vi "Configure Remote Terminal 2.vi"(8 "error in (no error)":errorcluster) -> (0 "error out":errorcluster, 3 "Remote Terminal":refnum<class "Remote Terminal.lvclass">)   [LabVIEW 2016, in "BCI-1553 RealTime API Examples.lvlib"]
uses:
  BCI-1553 RealTime API Examples.lvlib
  <vilib>/Bloomy/BCI-1553 Driver/RealTime/Remote Terminal/Remote Terminal.lvclass
  <vilib>/Bloomy/BCI-1553 Driver/RealTime/Frames & Messages/TypeDefs/Command Terminal Address.ctl
  <vilib>/Bloomy/BCI-1553 Driver/RealTime/Frames & Messages/TypeDefs/Command Type.ctl
  <vilib>/Bloomy/BCI-1553 Driver/RealTime/Frames & Messages/TypeDefs/Command SubAddress.ctl
  <vilib>/Bloomy/BCI-1553 Driver/RealTime/Frames & Messages/TypeDefs/Command Word Count.ctl
  <vilib>/Bloomy/BCI-1553 Driver/RealTime/Remote Terminal/TypeDefs/RT Configuration.ctl
  <vilib>/Bloomy/BCI-1553 Driver/RealTime/Remote Terminal/TypeDefs/RT-RT Timeout.ctl
  <vilib>/Bloomy/BCI-1553 Driver/RealTime/Remote Terminal/TypeDefs/Mode Code 17 Sync Configuration.ctl
  <vilib>/Bloomy/BCI-1553 Driver/RealTime/Remote Terminal/TypeDefs/RT Timetag Configuration.ctl
  <vilib>/Bloomy/BCI-1553 Driver/RealTime/BCI-1553 API.lvlib
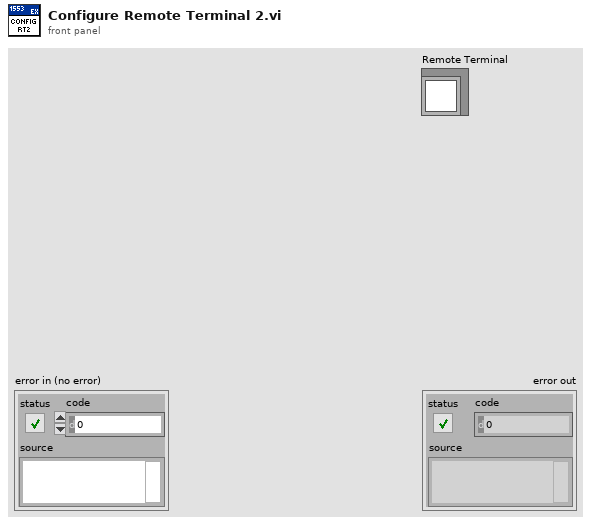
[diagram p1: front panel]
types:
  T1 = typedef "BCI-1553 API.lvlib/Remote Terminal.lvclass/RT Timetag Configuration.ctl" = enum16{"Disabled", "2us", "4us", "8us", "16us", "32us", "64us"}
  T2 = typedef "BCI-1553 API.lvlib/Remote Terminal.lvclass/RT-RT Timeout.ctl" = enum16{"57us", "62us", "100us", "180us"}
  T3 = typedef "BCI-1553 API.lvlib/Remote Terminal.lvclass/RT Configuration.ctl" = cluster{"RT-RT Timeout":T2, "Inhibit Bus A":bool, "Inhibit Bus B":bool, "Broadcast CMD Invalid":bool, "UnDef MCs Invalid":bool, "Notice 2 Data Storage":bool, "SMCP":bool, "Temp RX Buffer":bool, "Alt BIT Enable":bool, "Auto Bus Shutdown":bool, "MC 16 SR Reset":bool, "MC 17 Sync":T4, "MC 8 Reset":bool, "Remote Terminal Timetag Config":T1}
  T4 = typedef "BCI-1553 API.lvlib/Remote Terminal.lvclass/Mode Code 17 Sync Configuration.ctl" = enum16{"Sync if Bit 0 = 1", "Sync if Bit 0 = 0", "Sync Unconditionally"}
  T5 = typedef "BCI-1553 API.lvlib/Command Word Count.ctl" = enum16{"1", "2", "3", "4", "5", "6", "7", "8", "9", "10", "11", "12", "13", "14", "15", "16", "17", "18", "19", "20", "21", "22", "23", "24", "25", "26", "27", "28", "29", "30", "31", "32"}
  T6 = typedef "BCI-1553 API.lvlib/Command SubAddress.ctl" = enum16{"Mode Code", "1", "2", "3", "4", "5", "6", "7", "8", "9", "10", "11", "12", "13", "14", "15", "16", "17", "18", "19", "20", "21", "22", "23", "24", "25", "26", "27", "28", "29", "30"}
  T7 = typedef "BCI-1553 API.lvlib/Command Type.ctl" = enum16{"Transmit", "Receive"}
  T8 = typedef "BCI-1553 API.lvlib/Command Terminal Address.ctl" = enum16{"0", "1", "2", "3", "4", "5", "6", "7", "8", "9", "10", "11", "12", "13", "14", "15", "16", "17", "18", "19", "20", "21", "22", "23", "24", "25", "26", "27", "28", "29", "30", "Broadcast"}
  T9 = typedef "BCI-1553 API.lvlib/Remote Terminal.lvclass/RT Command Config.ctl" = cluster{"Command Type":T7, "SubAddress":T6, "Word Count\\Mode Code":T5, "Initial Data":u16[], "Data Fields":T10[]}
  T10 = typedef "BCI-1553 API.lvlib/Simplified Parameter Data Table.ctl" = cluster{"Parameter Name":string, "Base Word":u16, "Scaling Info":T11}
  T11 = typedef "BCI-1553 API.lvlib/Scaling Information.ctl" = cluster{"Bit Offset":i32, "Bit Count":i32, "LSB Resolution":dbl, "2's Complement":bool, "Big Endian":bool, "Sign Bit":bool}
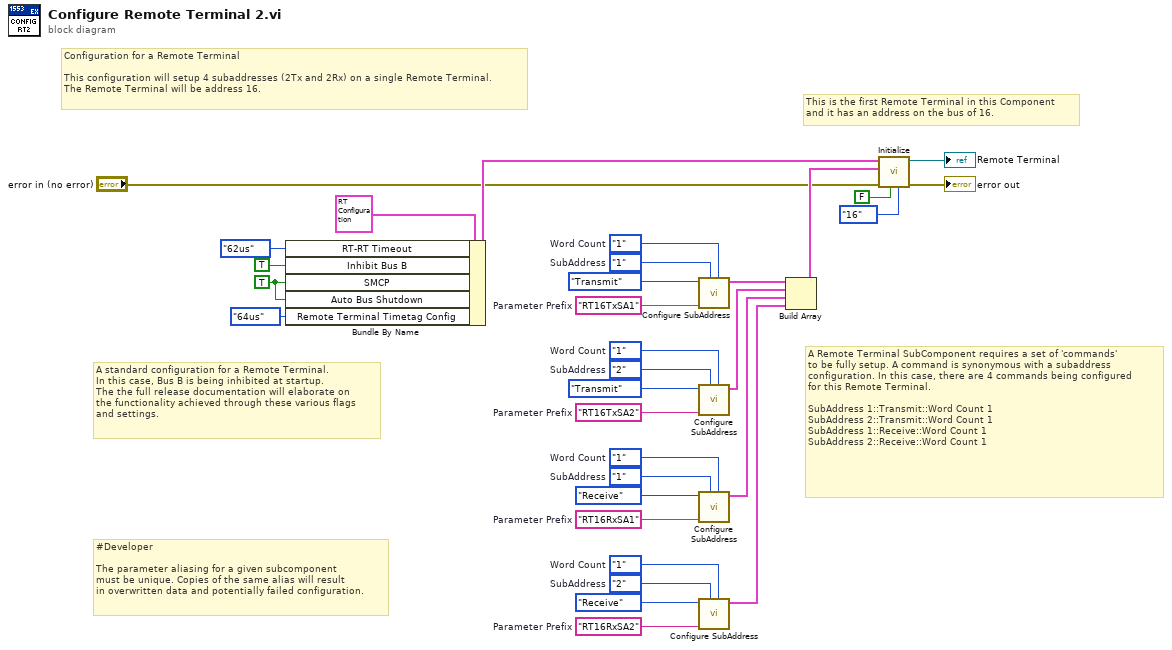
[diagram p0: block diagram]
diagram:
  w2 = TRUE ("SMCP")
  w16 = Command_Word_Count."1"  # Word Count
  w15 = Command_SubAddress."2"  # SubAddress
  w18 = Command_Word_Count."1"  # Word Count
  w17 = Command_SubAddress."1"  # SubAddress
  w19 = Command_Word_Count."1"  # Word Count
  w20 = Command_SubAddress."2"  # SubAddress
  w21 = "RT16RxSA2"  # Parameter Prefix
  w22 = "RT16RxSA1"  # Parameter Prefix
  w23 = "RT16TxSA2"  # Parameter Prefix
  w24 = "RT16TxSA1"  # Parameter Prefix
  w25 = Command_Word_Count."1"  # Word Count
  w26 = Command_SubAddress."1"  # SubAddress
  # "A Remote Terminal SubComponent requires a set of 'commands'\nto be fully setup. A command is synonymous with a subaddress\nconfiguration. In this case, there are 4 commands being configured\nfor this Remote Terminal.\n\nSubAddress 1::Transmit::Word Count 1\nSubAddress 2::Transmit::Word Count 1\nSubAddress 1::Receive::Word Count 1\nSubAddress 2::Receive::Word Count 1"
  # "A standard configuration for a Remote Terminal.\nIn this case, Bus B is being inhibited at startup.\nThe the full release documentation will elaborate on\nthe functionality achieved through these various flags\nand settings."
  # "#Developer\n\nThe parameter aliasing for a given subcomponent\nmust be unique. Copies of the same alias will result\nin overwritten data and potentially failed configuration."
  # "This is the first Remote Terminal in this Component\nand it has an address on the bus of 16."
  # "Configuration for a Remote Terminal\n\nThis configuration will setup 4 subaddresses (2Tx and 2Rx) on a single Remote Terminal.\nThe Remote Terminal will be address 16."
  n1 = Bundle By Name(cluster=T3 {"RT-RT Timeout"=enum."57us", "Inhibit Bus A"=FALSE, "Inhibit Bus B"=FALSE, "Broadcast CMD Invalid"=FALSE, "UnDef MCs Invalid"=FALSE, "Notice 2 Data Storage"=FALSE, "SMCP"=FALSE, "Temp RX Buffer"=FALSE, "Alt BIT Enable"=FALSE, "Auto Bus Shutdown"=FALSE, "MC 16 SR Reset"=FALSE, "MC 17 Sync"=enum."Sync if Bit 0 = 1", "MC 8 Reset"=FALSE, "Remote Terminal Timetag Config"=enum."Disabled"} ("RT Configuration"), "RT-RT Timeout"=RT-RT_Timeout."62us", "Inhibit Bus B"=TRUE, "SMCP"=w2, "Auto Bus Shutdown"=w2, "Remote Terminal Timetag Config"=RT_Timetag_Configuration."64us") -> (w8:T3)
  n2 = call "Configure SubAddress.vi"("Word Count\\Mode Code"=w25, "SubAddress"=w26, "Parameter Prefix"=w24, "Command Type"=Command_Type."Transmit") -> ("SubAddress Configuration"=w14:T9)  [unwired: 7 in]
  n3 = call "Configure SubAddress.vi"("Word Count\\Mode Code"=w19, "SubAddress"=w20, "Parameter Prefix"=w23, "Command Type"=Command_Type."Transmit") -> ("SubAddress Configuration"=w13:T9)  [unwired: 7 in]
  n4 = call "Configure SubAddress.vi"("Word Count\\Mode Code"=w18, "SubAddress"=w17, "Parameter Prefix"=w22, "Command Type"=Command_Type."Receive") -> ("SubAddress Configuration"=w12:T9)  [unwired: 7 in]
  n5 = call "Configure SubAddress.vi"("Word Count\\Mode Code"=w16, "SubAddress"=w15, "Parameter Prefix"=w21, "Command Type"=Command_Type."Receive") -> ("SubAddress Configuration"=w11:T9)  [unwired: 7 in]
  n6 = Build Array(w14, w13, w12, w11) -> (w10:T9[])
  n7 = call <vilib>:"Initialize.vi"("Terminal Address"=Command_Terminal_Address."16", "RT 1?"=FALSE, "error in (no error)"="error in (no error)", "RT Commands"=w10, "RT Configuration"=w8) -> ("error out"=→"error out":errorcluster, "Remote Terminal out"=→"Remote Terminal":refnum<class "Remote Terminal.lvclass">)  [unwired: 5 in]
